vi "Create Wheel Angular Velocity Row.vi"(8 "error in (no error)":errorcluster, 10 "steering angle (rad)":dbl, 11 "steering wheel in":refnum<class "NI_Robotics_Steering Wheel.lvclass">) -> (0 "error out":errorcluster, 2 "wheel angular velocity row":dbl[](array[numeric]), 3 "steering wheel out":refnum<class "NI_Robotics_Steering Wheel.lvclass">)   [LabVIEW 2017, in "NI_Robotics_Steering Wheel.lvclass"]
uses:
  <vilib>/robotics/Steering/Steering Wheel/NI_Robotics_Steering Wheel.lvclass
  c:/Program Files (x86)/National Instruments/LabVIEW 2017/vi.lib/robotics/Steering/Wheel/NI_Robotics_Wheel.lvclass
  <vilib>/robotics/Steering/Wheel/NI_Robotics_Wheel.lvclass/NI_Robotics_Wheel.ctl
  <vilib>/robotics/Steering/Wheel/NI_Robotics_Wheel.lvclass
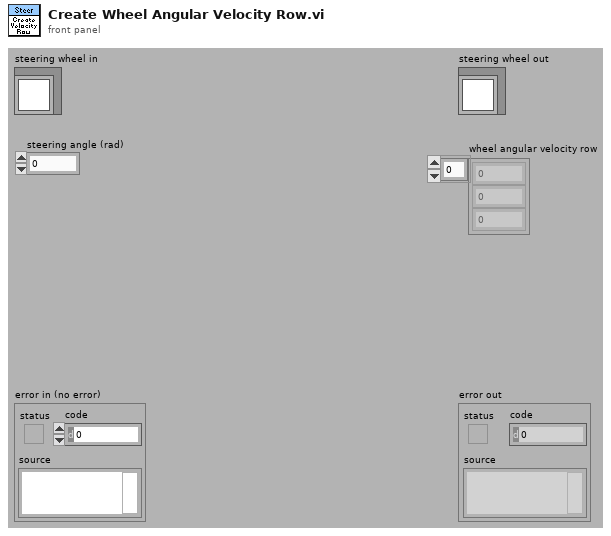
[diagram p1: front panel]
types:
  T1 = typedef "NI_Matrix.lvlib/RealMatrix.ctl" = dbl[][]
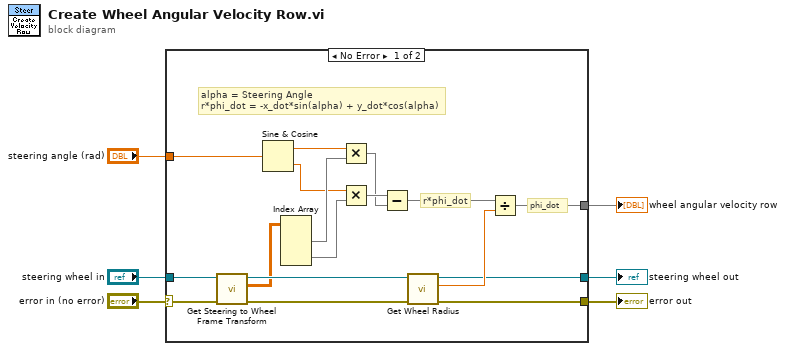
[diagram p0: block diagram]
diagram:
  n1 = case shown="No Error" "error in (no error)" {
    selector: "error in (no error)" -> [w12 w25]
    tunnel: [w16 w25] -> w5
    tunnel: "steering wheel in" -> [w14 w24]
    tunnel: [w17 w24] -> w3
    tunnel: "steering angle (rad)" -> [w9 _]
    tunnel: [w15 _] -> w1
    frame No Error {
      # "phi_dot"
      # "r*phi_dot"
      # "alpha = Steering Angle\nr*phi_dot = -x_dot*sin(alpha) + y_dot*cos(alpha)"
      n2 = call <vilib>:"Get Steering to Wheel Frame Transform.vi"("error in (no error)"=w12, "wheel in"=w14) -> ("error out"=w11:errorcluster, "steering to wheel frame transform"=w10:T1, "wheel out"=w13:refnum<class "NI_Robotics_Steering Wheel.lvclass">)  [unwired: 7 in]
      n3 = Sine & Cosine(0:w9) -> (1:w8:dbl, 2:w7:dbl)
      n4 = Index Array(array=w10) -> (element #1=w23:dbl[], element #2=w22:dbl[])  [unwired: 4 in]
      n5 = Multiply(x=w8, y=w23) -> (x*y=w20:dbl[])
      n6 = Multiply(x=w7, y=w22) -> (x*y=w21:dbl[])
      n7 = Subtract(x=w21, y=w20) -> (x-y=w19:dbl[])
      n8 = call <vilib>:"Get Wheel Radius.vi"("error in (no error)"=w11, "wheel in"=w13) -> ("error out"=w16:errorcluster, "wheel radius"=w18:dbl, "wheel out"=w17:refnum<class "NI_Robotics_Steering Wheel.lvclass">)  [unwired: 7 in]
      n9 = Divide(x=w19, y=w18) -> (x/y=w15:dbl[])
    }
    frame Error {
    }
  }
  "error out" <- w5
  "steering wheel out" <- w3
  "wheel angular velocity row" <- w1
